vi "SNTP Light RT Driver VI_SNTP Part_Offset_Filtering.vi"(9 "mean":dbl, 10 "Offset (s) in":dbl, 11 "Synchronized?":bool) -> (3 "Offset (s) out":dbl)   [LabVIEW 2013]
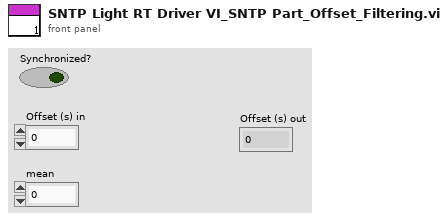
[diagram p1: front panel]
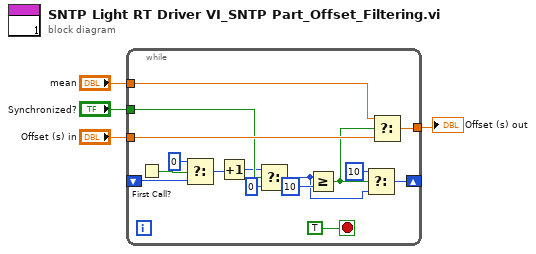
[diagram p0: block diagram]
diagram:
  n1 = while {
    tunnel: [w20] -> w4
    tunnel: "Offset (s) in" -> [w19]
    tunnel: "Synchronized?" -> [w14]
    tunnel: "mean" -> [w8]
    shift-right: [w7] -> _
    shift-left: _ -> [w16]
    stop <- TRUE stop-if-true
    n2 = First Call?() -> (First Call?: T/F=w17:bool)
    n3 = Select(t=u8 0, s=w17, f=w16) -> (s? t:f=w12:u8)
    n4 = Increment(x=w12) -> (x+1=w13:u8)
    n5 = Select(t=w13, s=w14, f=u8 0) -> (s? t:f=w5:u8)
    n6 = Greater Or Equal?(x=w5, y=u8 10) -> (x >= y?=w9:bool)
    n7 = Select(t=u8 10, s=w9, f=w5) -> (s? t:f=w7:u8)
    n8 = Select(t=w8, s=w9, f=w19) -> (s? t:f=w20:dbl)
  }
  "Offset (s) out" <- w4
